vi "initialise.vi"(8 "error in (no error)":errorcluster, 11 "GenericPlugin in":refnum<class "FPGAWrapperAN110607Galvo.lvclass">) -> (0 "error out":errorcluster, 3 "GenericPlugin out":refnum<class "FPGAWrapperAN110607Galvo.lvclass">)   [LabVIEW 2010, in "FPGAWrapperAN110607Galvo.lvclass"]
doc: "The dynamic dispatch-version of this VI initalises the plug-in object by allocating and initalising any dynamic resources need."
uses:
  FPGAWrapperAN110607Galvo.lvclass
  GenericFPGAWrapper/GenericFPGAWrapper/GenericFPGAWrapper.lvclass
  <vilib>/userDefined/High Color/nirio_resource_hc.ctl
  <vilib>/rvi/interface/nirviOpenFPGA/nirviOpenFPGA.xnode
  FPGA Bitfiles/main.lvbitx
  <vilib>/rvi/ClientSDK/nirviWhatTheDeviceIsDoing.ctl
  <vilib>/rvi/interface/nirviMethod/nirviMethod.xnode
  <vilib>/rvi/interface/nirviReadWriteControl/nirviReadWriteControl.xnode
  <vilib>/rvi/interface/common/niFpgaNodeNameForErrorReporting.ctl
  <vilib>/rvi/errors/niLvFpgaWhatHappensToTopLevelVI.ctl
  <vilib>/FPGAPlugInAG/PXIe-7962R/niLvFpga_Open_PXIe-7962R.vi
  <vilib>/rvi/interface/common/dynamic/niFpgaDynamicAddResources.vi
  <vilib>/FPGAPlugInAG/Dynamic/niLvFpga_Reset_Dynamic.vi
  <vilib>/Utility/error.llb/Error Cluster From Error Code.vi
  <vilib>/rvi/errors/niLvFpgaAdjustHostInterfaceError.vi
  NiFpgaLv.dll
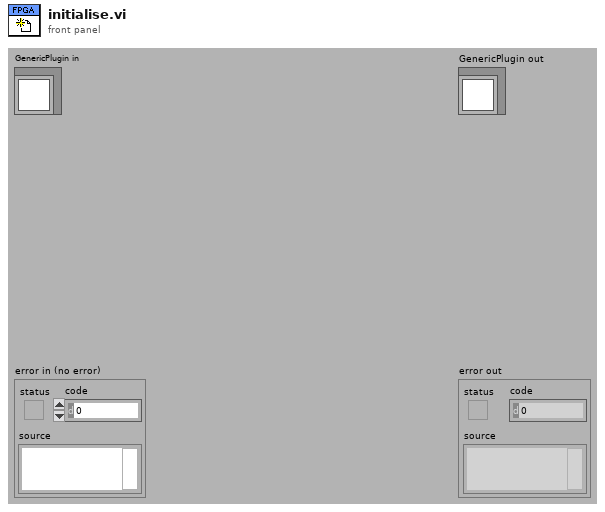
[diagram p1: front panel]
types:
  T1 = typedef "nirio_resource_hc.ctl" = tag
  T2 = typedef "niFpgaNodeNameForErrorReporting.ctl" = enum16{"Open FPGA VI Reference", "Read/Write Control", "Invoke Method: Abort", "Invoke Method: Acknowledge IRQ", "Invoke Method: Download", "Invoke Method: FIFO.Configure", "Invoke Method: FIFO.Read", "Invoke Method: FIFO.Start", "Invoke Method: FIFO.Stop", "Invoke Method: FIFO.Write", "Invoke Method: Reset", "Invoke Method: Run", "Invoke Method: Wait on IRQ", "Close FPGA VI Reference"}
  T3 = typedef "niLvFpgaWhatHappensToTopLevelVI.ctl" = enum16{"top level VI scripted behind XNode", "top level VI inlined behind XNode"}
  T4 = typedef "nirviWhatTheDeviceIsDoing.ctl" = enum32{"nothing", "something other than LabVIEW FPGA", "FPGA interface", "interactive", "emulation"}
  T5 = typedef "FPGAWrapperAN110607Galvo.lvclass/FPGA_VI_ref.ctl" = refnum<k20>
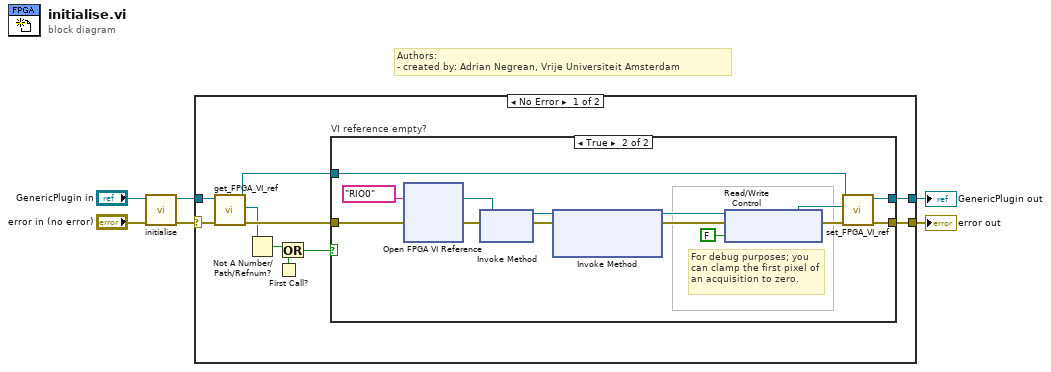
[diagram p0: block diagram]
diagram:
  # "Authors: \n- created by: Adrian Negrean, Vrije Universiteit Amsterdam"
  n1 = call-parent "initialise.vi"("error in (no error)"="error in (no error)", "GenericPlugin in"="GenericPlugin in") -> ("error out"=w1:errorcluster, "GenericPlugin out"=w3:refnum<class "FPGAWrapperAN110607Galvo.lvclass">)  [unwired: 8 in]
  n2 = case shown="No Error" w1 {
    selector: w1 -> [w13 w173]
    tunnel: [w11 w173] -> w6
    tunnel: w3 -> [w14 w172]
    tunnel: [w10 w172] -> w5
    frame No Error {
      n3 = call-dynamic "get_FPGA_VI_ref.vi"("error in (no error)"=w13, "FPGAWrapperAN110607Galvo in"=w14) -> ("error out"=w16:errorcluster, "FPGA VI reference"=w9:T5, "FPGAWrapperAN110607Galvo out"=w12:refnum<class "FPGAWrapperAN110607Galvo.lvclass">)  [unwired: 7 in]
      n4 = Not A Number/Path/Refnum?(number/path/refnum=w9) -> (NaN/Path/Refnum?=w8:bool)
      n5 = First Call?() -> (First Call?: T/F=w7:bool)
      n6 = Or(x=w8, y=w7) -> (x .or. y?=w15:bool)
      n7 = case "VI reference empty?" shown="True" w15 {
        tunnel: w16 -> [w17 w31]
        tunnel: w12 -> [w18 w27]
        tunnel: [w17 w29] -> w11
        tunnel: [w18 w28] -> w10
        frame False {
        }
        frame True {
          # "For debug purposes; you can clamp the first pixel of an acquisition to zero."
          n8 = xnode "Open FPGA VI Reference"("error in"=w31, "resource name"=T1 "RIO0") -> ("FPGA VI Reference Out"=w24:refnum<k20>, "error out"=w30:errorcluster)
          n9 = xnode "Invoke Method"("FPGA VI Reference In"=w24, "error in"=w30) -> ("FPGA VI Reference Out"=w25:refnum<k20>, "error out"=w26:errorcluster)
          n10 = xnode "Invoke Method"("FPGA VI Reference In"=w25, "error in"=w26) -> ("FPGA VI Reference Out"=w21:refnum<k20>, "error out"=w23:errorcluster)  [unwired: 1 in]
          n11 = xnode "Read/Write Control"("FPGA VI Reference In"=w21, "error in"=w23, "clamp first pixel?"=FALSE) -> ("FPGA VI Reference Out"=w20:refnum<k20>, "error out"=w22:errorcluster)
          n12 = call-dynamic "set_FPGA_VI_ref.vi"("error in (no error)"=w22, "FPGA VI reference"=w20, "FPGAWrapperAN110607Galvo in"=w27) -> ("error out"=w29:errorcluster, "FPGAWrapperAN110607Galvo out"=w28:refnum<class "FPGAWrapperAN110607Galvo.lvclass">)  [unwired: 7 in]
        }
      }
    }
    frame Error {
    }
  }
  "error out" <- w6
  "GenericPlugin out" <- w5
